vi "Stackingsetpointsvi.vi"(11 "Robot Controls":T2) -> ()   [LabVIEW 2014]
uses:
  Robot Commands.ctl
  Global Variables/Refnum Names.vi
panel:
  in  "Test Setpoints":T1
  out "Pos1 5":bool
  out "Pos1 4":bool
  out "Pos1 3":bool
  out "Pos1 2":bool
  out "Pos1":bool
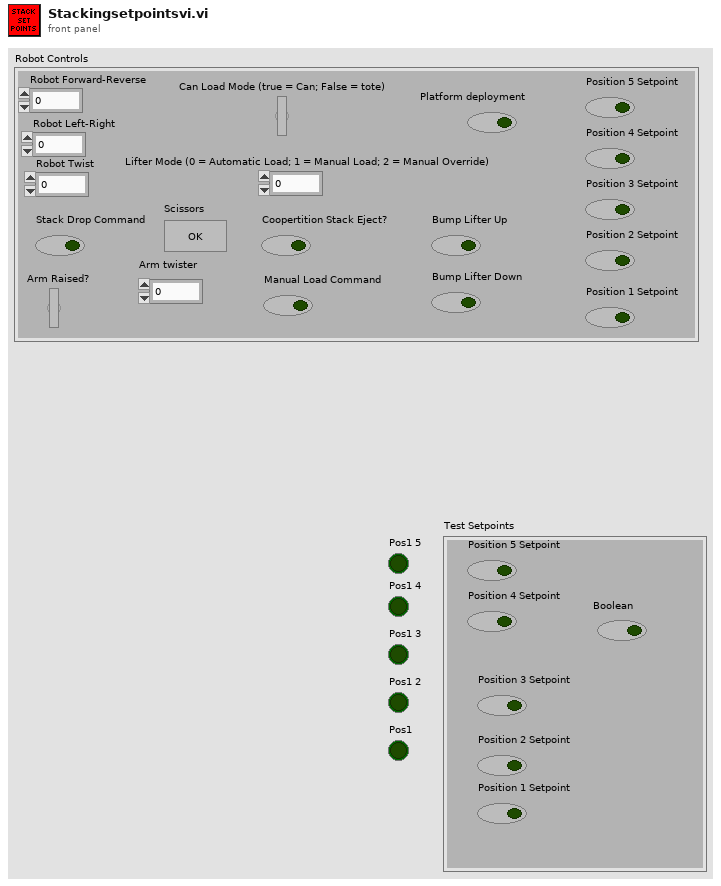
[diagram p1: front panel]
types:
  T1 = cluster{"Position 1 Setpoint":bool, "Position 2 Setpoint":bool, "Position 3 Setpoint":bool, "Position 4 Setpoint":bool, "Position 5 Setpoint":bool, "Boolean":bool}
  T2 = typedef "Robot Commands.ctl" = cluster{"Robot Forward-Reverse":dbl, "Robot Left-Right":dbl, "Robot Twist":dbl, "Can Load Mode (true = Can; False = tote)":bool, "Lifter Mode (0 = Automatic Load; 1 = Manual Load; 2 = Manual Override)":dbl, "Stack Drop Command":bool, "Arm Raised?":bool, "Coopertition Stack Eject?":bool, "Position 1 Setpoint":bool, "Position 2 Setpoint":bool, "Position 3 Setpoint":bool, "Position 4 Setpoint":bool, "Position 5 Setpoint":bool, "Bump Lifter Down":bool, "Bump Lifter Up":bool, "Manual Load Command":bool, "Arm twister":dbl, "Scissors":bool, "Platform deployment":bool}
  T3 = typedef "WPI_MotorControlDeviceRef.ctl" = cluster{"DeviceStatus":errorcluster, "Type":T4, "PWM":cluster{"Controller":T5, "PWM Channel":T6, "DeadBand":T7}, "CAN":cluster{"Device Number":u8, "Control Mode":T8, "Semaphore":T9, "Max Vout":dbl, "TalonSRX Control Mode":T10}, "Invert":bool, "TransformRef":T11, "InvTransformRef":T11}
  T4 = typedef "WPI_MotorControlType.ctl" = enum16{"PWM", "CAN", "CANTalonSRX"}
  T5 = typedef "FPGA_TypedefDigitalModule.ctl" = enum16{"Controller 1"}
  T6 = typedef "FPGA_DIOPWMChannel.ctl" = enum8{"PWM 0", "PWM 1", "PWM 2", "PWM 3", "PWM 4", "PWM 5", "PWM 6", "PWM 7", "PWM 8", "PWM 9", "PWM MXP 0", "PWM MXP 1", "PWM MXP 2", "PWM MXP 3", "PWM MXP 4", "PWM MXP 5", "PWM MXP 6", "PWM MXP 7", "PWM MXP 8", "PWM MXP 9", "Invalid"}
  T7 = typedef "WPI_PWMDeadband.ctl" = cluster{"Name":string, "maxPositivePwm":i32, "minPositivePwm":i32, "centerPwm":i32, "maxNegativePwm":i32, "minNegativePwm":i32, "angularRange":u16}
  T8 = typedef "WPI_CANJaguar_ControlMode.ctl" = enum8{"Percent VBus", "Current", "Speed", "Position", "Voltage"}
  T9 = typedef "Semaphore RefNum" = refnum<k1>
  T10 = typedef "WPI_CANTalonSRX_APIControlMode.ctl" = enum8{"Percent VBus", "Speed", "Position", "Slave", "Unchanged / Invalid"}
  T11 = typedef "WPI_PWMTransform_ConPane.ctl" = refnum<vi>
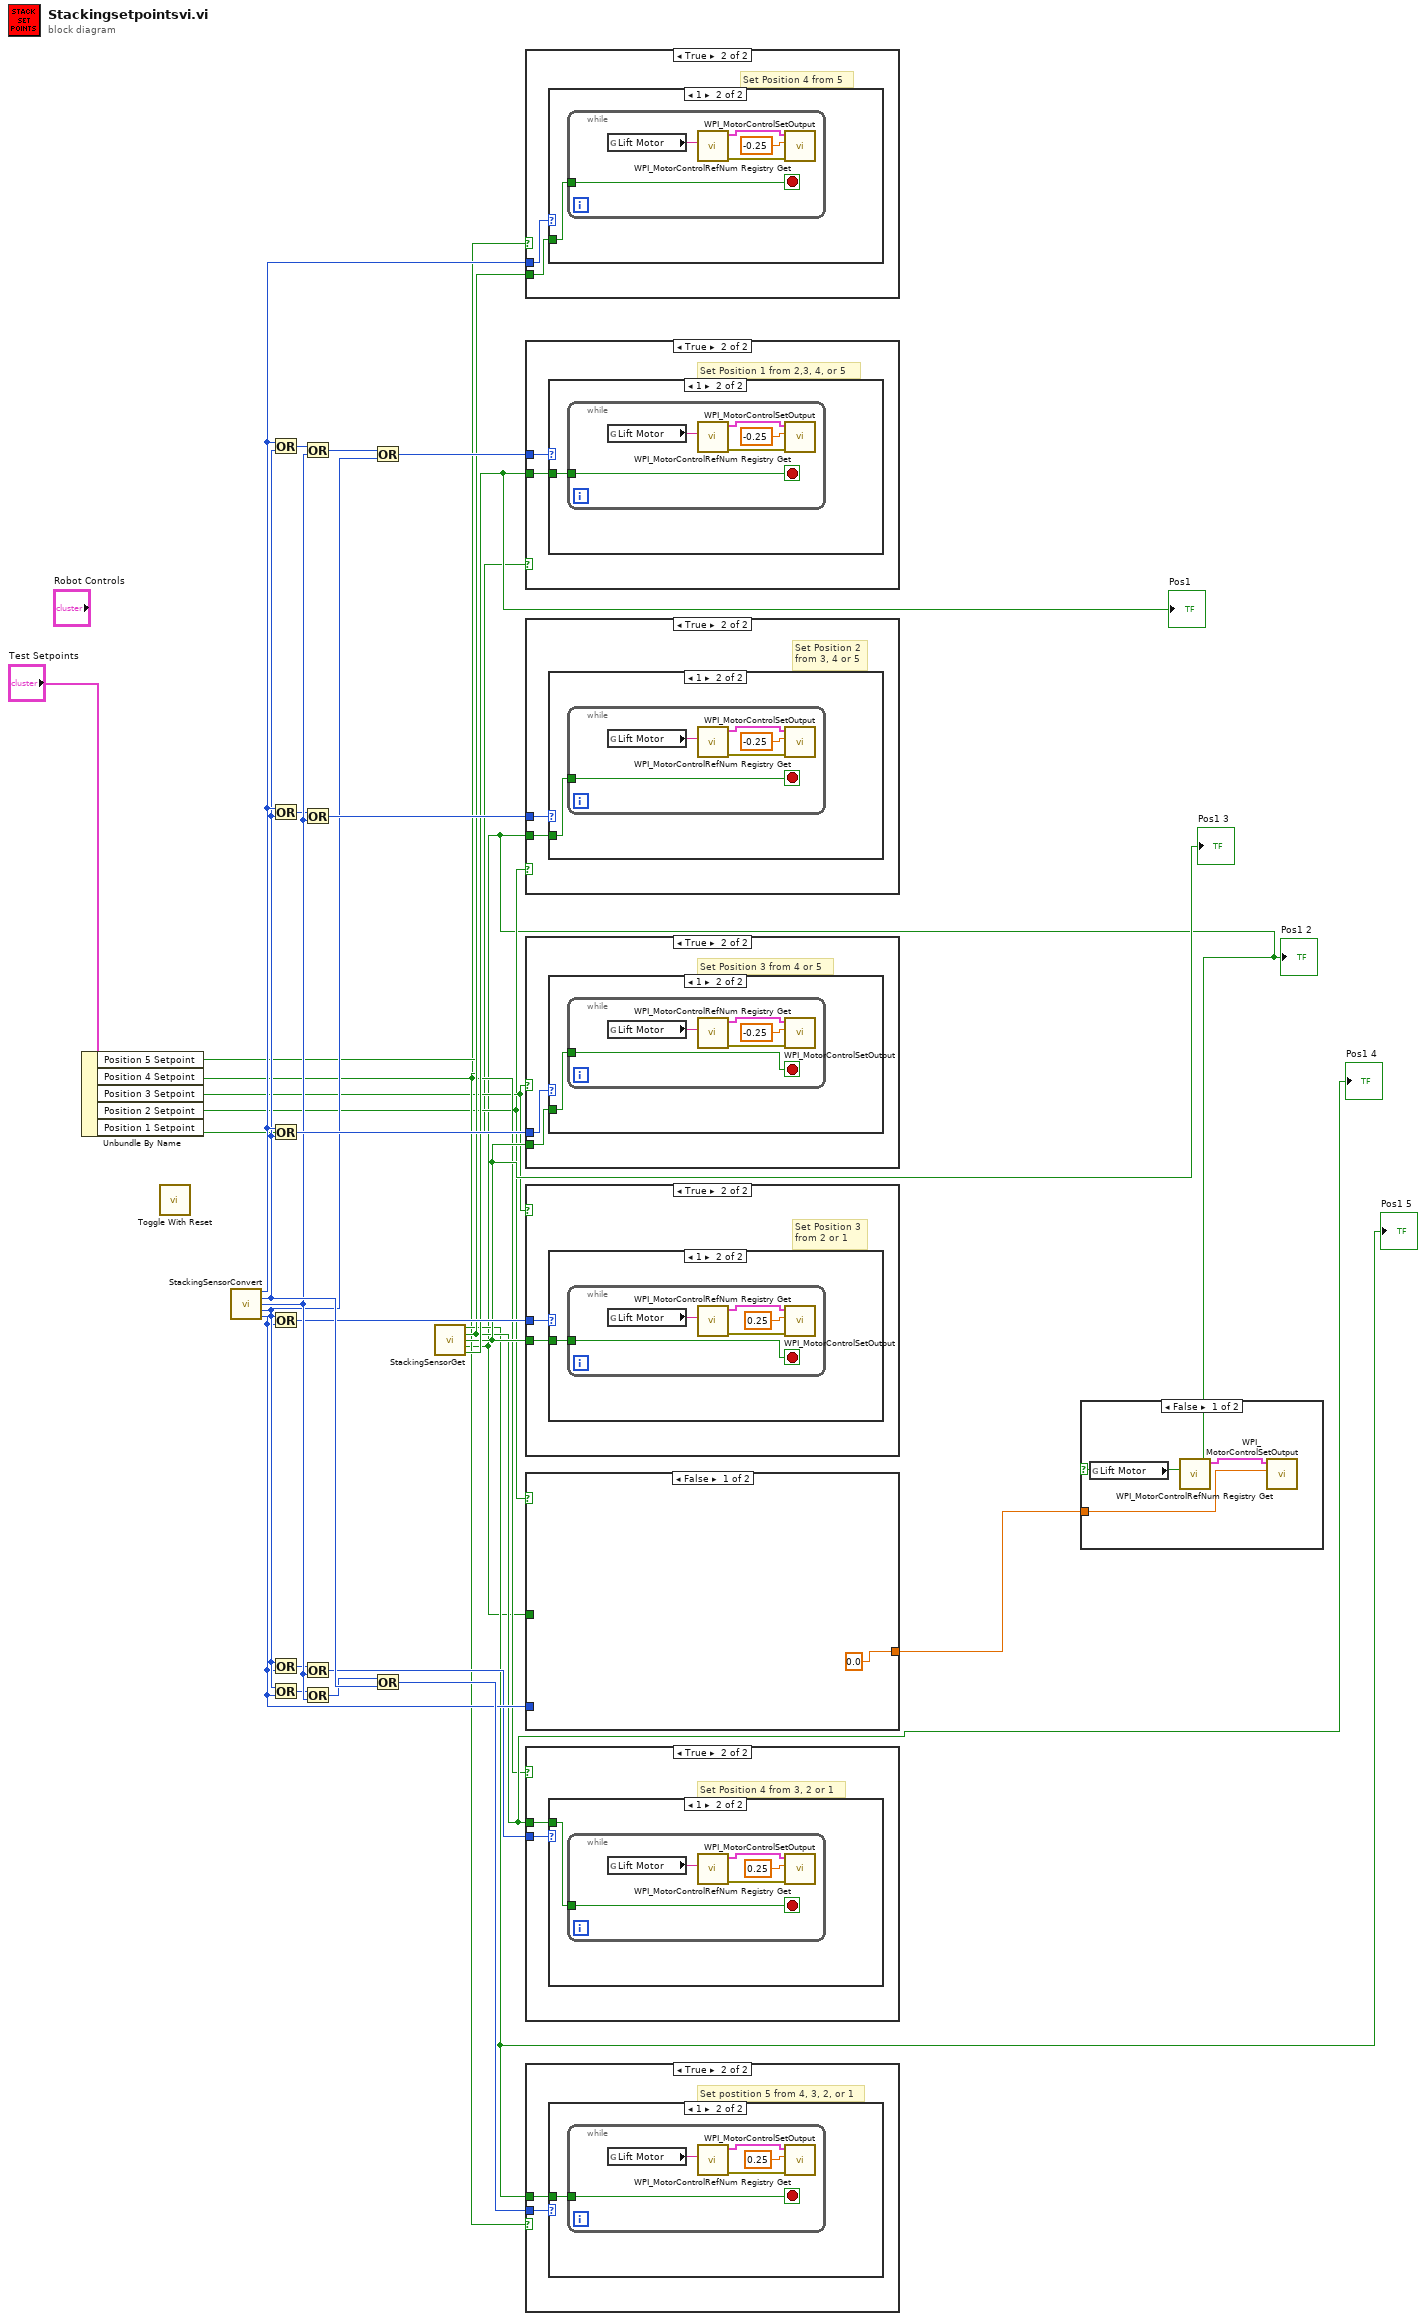
[diagram p0: block diagram]
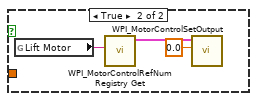
[diagram p2: hidden frame]
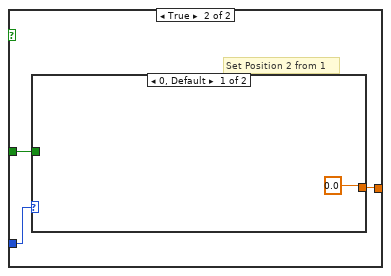
[diagram p17: hidden frame]
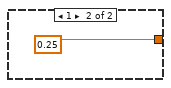
[diagram p18: hidden frame]
diagram:
  n1 = Unbundle By Name("Test Setpoints") -> ("Position 5 Setpoint"=w7:bool, "Position 4 Setpoint"=w6:bool, "Position 3 Setpoint"=w5:bool, "Position 2 Setpoint"=w4:bool, "Position 1 Setpoint"=w3:bool)
  n2 = call "Toggle With Reset.vi"() -> ()  [unwired: 2 in, 1 out]
  n3 = call "StackingSensorConvert.vi"() -> ("Pos5"=w29:u32, "Pos4"=w27:u32, "Pos3"=w25:u32, "Pos2"=w22:u32, "Pos1"=w18:u32)  [unwired: 11 in]
  n4 = Or(x=w29, y=w27) -> (x .or. y?=w21:u32)
  n5 = Or(x=w29, y=w27) -> (x .or. y?=w24:u32)
  n6 = Or(x=w29, y=w27) -> (x .or. y?=w28:u32)
  n7 = Or(x=w22, y=w18) -> (x .or. y?=w13:u32)
  n8 = Or(x=w22, y=w18) -> (x .or. y?=w14:u32)
  n9 = Or(x=w22, y=w18) -> (x .or. y?=w16:u32)
  n10 = Or(x=w21, y=w25) -> (x .or. y?=w20:u32)
  n11 = Or(x=w24, y=w25) -> (x .or. y?=w26:u32)
  n12 = Or(x=w14, y=w25) -> (x .or. y?=w15:u32)
  n13 = Or(x=w16, y=w25) -> (x .or. y?=w17:u32)
  n14 = Or(x=w20, y=w22) -> (x .or. y?=w23:u32)
  n15 = Or(x=w17, y=w27) -> (x .or. y?=w19:u32)
  n16 = call "StackingSensorGet.vi"() -> ("Pos5"=w9:bool, "Pos4"=w10:bool, "Pos3"=w11:bool, "Pos2"=w2:bool, "Pos1"=w12:bool)  [unwired: 10 in, 1 out]
  "Pos1" <- w12
  "Pos1 2" <- w2
  "Pos1 5" <- w9
  "Pos1 3" <- w11
  "Pos1 4" <- w10
  n17 = case shown="True" w6 {
    tunnel: w29 -> [_ w31]
    tunnel: w10 -> [_ w30]
    frame False {
    }
    frame True {
      # "Set Position 4 from 5"
      n18 = case shown="1" w31 {
        tunnel: w30 -> [_ w32]
        frame 0, Default {
        }
        frame 1 {
          n19 = while {
            tunnel: w32 -> [w33]
            stop <- w33 stop-if-true
            n20 = global read "Refnum Names.vi" "Lift Motor"() -> (w35:string)
            n21 = call <vilib>:"WPI_MotorControlRefNum Registry Get.vi"("refnum name"=w35) -> ("error out"=w37:errorcluster, "MotorControlDevRef"=w36:T3)  [unwired: 9 in]
            n22 = call <vilib>:"WPI_MotorControlSetOutput.vi"("error in (no error)"=w37, "Output"=-0.25, "MotorControlDevRef"=w36) -> ()  [unwired: 6 in, 3 out]
          }
        }
      }
    }
  }
  n23 = case shown="True" w3 {
    tunnel: w12 -> [_ w39]
    tunnel: w23 -> [_ w38]
    frame False {
    }
    frame True {
      # "Set Position 1 from 2,3, 4, or 5"
      n24 = case shown="1" w38 {
        tunnel: w39 -> [_ w40]
        frame 0, Default {
        }
        frame 1 {
          n25 = while {
            tunnel: w40 -> [w41]
            stop <- w41 stop-if-true
            n26 = global read "Refnum Names.vi" "Lift Motor"() -> (w43:string)
            n27 = call <vilib>:"WPI_MotorControlRefNum Registry Get.vi"("refnum name"=w43) -> ("error out"=w45:errorcluster, "MotorControlDevRef"=w44:T3)  [unwired: 9 in]
            n28 = call <vilib>:"WPI_MotorControlSetOutput.vi"("error in (no error)"=w45, "Output"=-0.25, "MotorControlDevRef"=w44) -> ()  [unwired: 6 in, 3 out]
          }
        }
      }
    }
  }
  n29 = case shown="True" w4 {
    tunnel: w26 -> [_ w47]
    tunnel: w2 -> [_ w46]
    frame False {
    }
    frame True {
      # "Set Position 2 from 3, 4 or 5"
      n30 = case shown="1" w47 {
        tunnel: w46 -> [_ w48]
        frame 0, Default {
        }
        frame 1 {
          n31 = while {
            tunnel: w48 -> [w49]
            stop <- w49 stop-if-true
            n32 = global read "Refnum Names.vi" "Lift Motor"() -> (w51:string)
            n33 = call <vilib>:"WPI_MotorControlRefNum Registry Get.vi"("refnum name"=w51) -> ("error out"=w53:errorcluster, "MotorControlDevRef"=w52:T3)  [unwired: 9 in]
            n34 = call <vilib>:"WPI_MotorControlSetOutput.vi"("error in (no error)"=w53, "Output"=-0.25, "MotorControlDevRef"=w52) -> ()  [unwired: 6 in, 3 out]
          }
        }
      }
    }
  }
  n35 = case shown="True" w5 {
    tunnel: w28 -> [_ w55]
    tunnel: w11 -> [_ w54]
    frame False {
    }
    frame True {
      # "Set Position 3 from 4 or 5"
      n36 = case shown="1" w55 {
        tunnel: w54 -> [_ w56]
        frame 0, Default {
        }
        frame 1 {
          n37 = while {
            tunnel: w56 -> [w57]
            stop <- w57 stop-if-true
            n38 = global read "Refnum Names.vi" "Lift Motor"() -> (w59:string)
            n39 = call <vilib>:"WPI_MotorControlRefNum Registry Get.vi"("refnum name"=w59) -> ("error out"=w61:errorcluster, "MotorControlDevRef"=w60:T3)  [unwired: 9 in]
            n40 = call <vilib>:"WPI_MotorControlSetOutput.vi"("error in (no error)"=w61, "Output"=-0.25, "MotorControlDevRef"=w60) -> ()  [unwired: 6 in, 3 out]
          }
        }
      }
    }
  }
  n41 = case shown="True" w5 {
    tunnel: w13 -> [_ w63]
    tunnel: w11 -> [_ w62]
    frame False {
    }
    frame True {
      # "Set Position 3 from 2 or 1"
      n42 = case shown="1" w63 {
        tunnel: w62 -> [_ w64]
        frame 0, Default {
        }
        frame 1 {
          n43 = while {
            tunnel: w64 -> [w65]
            stop <- w65 stop-if-true
            n44 = global read "Refnum Names.vi" "Lift Motor"() -> (w67:string)
            n45 = call <vilib>:"WPI_MotorControlRefNum Registry Get.vi"("refnum name"=w67) -> ("error out"=w69:errorcluster, "MotorControlDevRef"=w68:T3)  [unwired: 9 in]
            n46 = call <vilib>:"WPI_MotorControlSetOutput.vi"("error in (no error)"=w69, "Output"=0.25, "MotorControlDevRef"=w68) -> ()  [unwired: 6 in, 3 out]
          }
        }
      }
    }
  }
  n47 = case shown="False" w4 {
    tunnel: w18 -> [_ w73]
    tunnel: w2 -> [_ w72]
    tunnel: [0.0 w71] -> w1
    frame False {
    }
    frame True {
      # "Set Position 2 from 1"
      n48 = case shown="0, Default" w73 {
        tunnel: w72 -> [_ _]
        tunnel: [0.0 0.25] -> w71
        frame 0, Default {
        }
        frame 1 {
        }
      }
    }
  }
  n49 = case shown="True" w6 {
    tunnel: w15 -> [_ w77]
    tunnel: w10 -> [_ w76]
    frame False {
    }
    frame True {
      # "Set Position 4 from 3, 2 or 1"
      n50 = case shown="1" w77 {
        tunnel: w76 -> [_ w78]
        frame 0, Default {
        }
        frame 1 {
          n51 = while {
            tunnel: w78 -> [w79]
            stop <- w79 stop-if-true
            n52 = global read "Refnum Names.vi" "Lift Motor"() -> (w81:string)
            n53 = call <vilib>:"WPI_MotorControlRefNum Registry Get.vi"("refnum name"=w81) -> ("error out"=w83:errorcluster, "MotorControlDevRef"=w82:T3)  [unwired: 9 in]
            n54 = call <vilib>:"WPI_MotorControlSetOutput.vi"("error in (no error)"=w83, "Output"=0.25, "MotorControlDevRef"=w82) -> ()  [unwired: 6 in, 3 out]
          }
        }
      }
    }
  }
  n55 = case shown="True" w7 {
    tunnel: w19 -> [_ w85]
    tunnel: w9 -> [_ w84]
    frame False {
    }
    frame True {
      # "Set postition 5 from 4, 3, 2, or 1"
      n56 = case shown="1" w85 {
        tunnel: w84 -> [_ w86]
        frame 0, Default {
        }
        frame 1 {
          n57 = while {
            tunnel: w86 -> [w87]
            stop <- w87 stop-if-true
            n58 = global read "Refnum Names.vi" "Lift Motor"() -> (w89:string)
            n59 = call <vilib>:"WPI_MotorControlRefNum Registry Get.vi"("refnum name"=w89) -> ("error out"=w91:errorcluster, "MotorControlDevRef"=w90:T3)  [unwired: 9 in]
            n60 = call <vilib>:"WPI_MotorControlSetOutput.vi"("error in (no error)"=w91, "Output"=0.25, "MotorControlDevRef"=w90) -> ()  [unwired: 6 in, 3 out]
          }
        }
      }
    }
  }
  n61 = case shown="False" w2 {
    tunnel: w1 -> [w92 _]
    frame False {
      n62 = global read "Refnum Names.vi" "Lift Motor"() -> (w93:string)
      n63 = call <vilib>:"WPI_MotorControlRefNum Registry Get.vi"("refnum name"=w93) -> ("MotorControlDevRef"=w94:T3)  [unwired: 9 in, 1 out]
      n64 = call <vilib>:"WPI_MotorControlSetOutput.vi"("Output"=w92, "MotorControlDevRef"=w94) -> ()  [unwired: 7 in, 3 out]
    }
    frame True {
      n65 = global read "Refnum Names.vi" "Lift Motor"() -> (w97:string)
      n66 = call <vilib>:"WPI_MotorControlRefNum Registry Get.vi"("refnum name"=w97) -> ("MotorControlDevRef"=w96:T3)  [unwired: 9 in, 1 out]
      n67 = call <vilib>:"WPI_MotorControlSetOutput.vi"("Output"=0.0, "MotorControlDevRef"=w96) -> ()  [unwired: 7 in, 3 out]
    }
  }
